vi "graphtoboolean.vi"(11 "Array in":i32[][](array[numeric])) -> (3 "Array out":bool[][](array[boolean]))   [LabVIEW 2016]
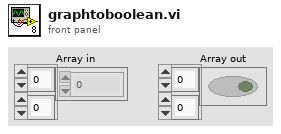
[diagram p1: front panel]
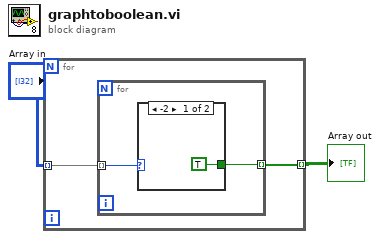
[diagram p0: block diagram]
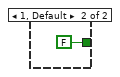
[diagram p2: hidden frame]
diagram:
  n1 = for {
    tunnel: "Array in" -> [w4] mode=indexing
    tunnel: [w3] -> w1 mode=indexing
    n2 = for {
      tunnel: w4 -> [w6] mode=indexing
      tunnel: [w5] -> w3 mode=indexing
      n3 = case shown="-2" w6 {
        tunnel: [TRUE FALSE] -> w5
        frame -2 {
        }
        frame 1, Default {
        }
      }
    }
  }
  "Array out" <- w1
